vi "Breakdown Point Detection.vi"() -> ()   [LabVIEW 2023]
doc: "This example shows the application of the continuous wavelet transform (CWT) in detecting breakdown points in a signal.\n\nBoth breakdown points and noise can generate large values in the resulting CWT coefficients. Breakdown points generate large positive or negative coefficients at all scales. Noise generates positive coefficients at some scales and negative coefficients at other scales. If you accumulate the coefficients at all scales, the coefficients of breakdown points are enlarged while the coefficients of noise at different scales counteract one another. Therefore, the peaks in the accumulated CWT coefficients correspond only to the breakdown points.\n\nThis example uses the WA Continuous Wavelet Transform VI to compute the CWT coefficients of a simulated signal and use the WA Multiscale Peak Detection VI to detect the peaks in the accumulated CWT coefficients.\n\n<b>Instructions:</b>\n1) Run this VI.\n2) Observe the peaks in the <b>CWT Coefficients Cumulation</b> graph.\n3) Browse the Block Diagram of this example to learn how to detect breakdown points in a signal with the continuous wavelet transform."
uses:
  <vilib>/addons/Wavelet Analysis/typedefs.llb/WA Data.ctl
  <vilib>/addons/Wavelet Analysis/continuous wavelet transform.llb/WA Continuous Wavelet Transform (Array).vi
  <vilib>/addons/Wavelet Analysis/application.llb/WA Multiscale Peak Detection (Array).vi
  <vilib>/addons/_Advanced Signal Processing/NI_AdvSigProcWA.lvlib
  <vilib>/Analysis/NI_AALBase.lvlib
panel:
  in  "stop":bool
  out "CWT Coefficients Cumulation":dbl[](graph)
  out "Breakdown locations":dbl[](array[numeric])
  in  "Noise level":dbl=0.4 min=0.0 step=0.05
  in  "Scales":i32=20 min=2 max=32 step=1
  out "Scalogram":dbl[][](graph)
  out "Signal":dbl[][](graph)
  # "Overview: Shows the application of the continuous wavelet transform (CWT) in detecting breakdown points in a signal.\nRequirements: LabVIEW Full Development System, Advanced Signal Processing Toolkit\nInstructions: \n1. Run this VI.\n2. Observe the peaks in the CWT Coefficients Cumulation graph.\n3. Browse the block diagram of this example to learn how to detect breakdown points in a signal with the continuous wavelet transform.\n4. Click Stop to stop the VI."
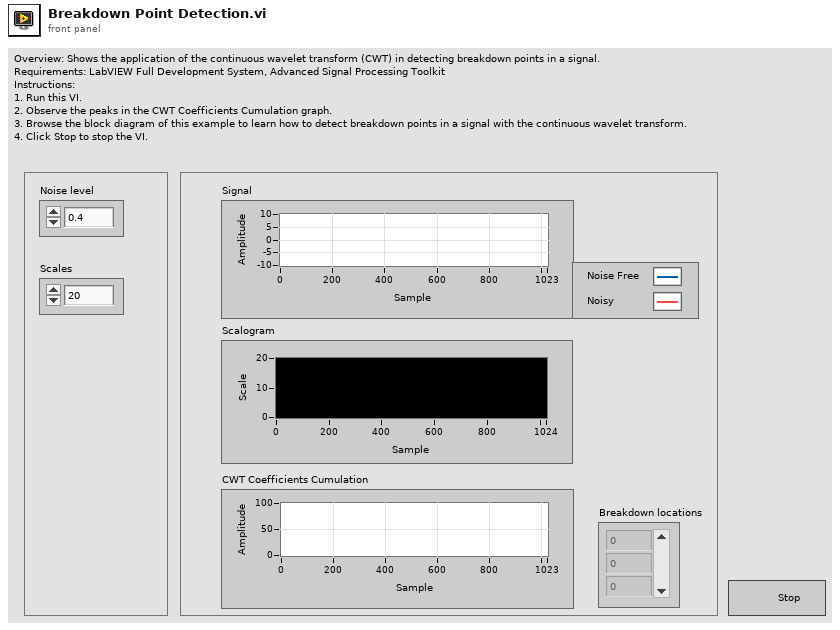
[diagram p1: front panel]
types:
  T1 = typedef "NI_AdvSigProcWA.lvlib/WA Data.ctl" = u16
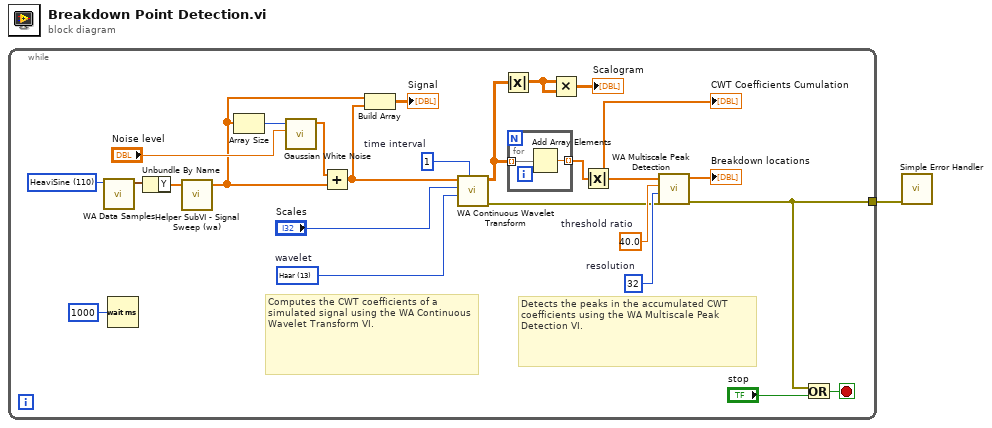
[diagram p0: block diagram]
diagram:
  n1 = while {
    tunnel: [w2] -> w1
    stop <- w10 stop-if-true
    w3 = T1 110 items=["1D Example Data"=100, "-"=101, "Doppler"=102, "HOP"=103, "TF Sine"=104, "Noisy Doppler"=105, "Sea Temperature"=106, "Sp500"=107, "Power Line"=108, "Engine Knocking"=109, "HeaviSine"=110, "Bumps"=111, "Blocks"=112, "Piece Regular"=113, "HypChirps"=114, "LinChirps"=115, "Chirps"=116, "Piece Polynomial"=117, "ECG"=131, "-"=118, "2D Example Data"=119, "-"=120, "Finger Print (Image)"=121, "Iris Flower (Image)"=122, "Mammogram (Image)"=123, "Lake (Image)"=127, "Two Can 1 (Image)"=132, "Two Can 2 (Image)"=133, "Camera Man (Image)"=134] ("data")
    w13 = u16 13 items=["Mexican Hat"=50, "Meyr"=51, "Morlet"=52, "-"=53, "db02"=0, "db03"=1, "db04"=2, "db05"=3, "db06"=4, "db07"=5, "db08"=6, "db09"=7, "db10"=8, "db11"=9, "db12"=10, "db13"=11, "db14"=12, "Haar"=13, "bior1_3"=14, "bior1_5"=15, "bior2_2"=16, "bior2_4"=17, "bior2_6"=18, "bior2_8"=19, "bior3_1"=20, "bior3_3"=21, "bior3_5"=22, "bior3_7"=23, "bior3_9"=24, "bior4_4 (FBI)"=25, "bior5_5"=38, "bior6_8"=39, "coif1"=26, "coif2"=27, "coif3"=28, "coif4"=29, "coif5"=30, "sym2"=31, "sym3"=32, "sym4"=33, "sym5"=34, "sym6"=35, "sym7"=36, "sym8"=37]  # wavelet
    w15 = 32  # resolution
    w16 = 40.0  # threshold ratio
    w25 = 1  # time interval
    # "Detects the peaks in the accumulated CWT coefficients using the WA Multiscale Peak Detection VI."
    # "Computes the CWT coefficients of a simulated signal using the WA Continuous Wavelet Transform VI."
    n2 = call <vilib>:"WA Data Samples.vi"("data"=w3) -> ("signal"=w26:waveform(dbl))  [unwired: 10 out]
    n3 = Wait (ms)(milliseconds to wait=u32 1000 ("millisecond multiple")) -> ()  [unwired: 1 out]
    n4 = Unbundle By Name(w26) -> ("Y"=w8:dbl[])
    n5 = call "Helper SubVI - Signal Sweep (wa).vi"("Signal in"=w8) -> ("Signal out"=w7:dbl[])  [unwired: 10 in]
    n6 = Array Size(array=w7) -> (size(s)=w23:i32)
    n7 = call <vilib>:"Gaussian White Noise.vi"("standard deviation"="Noise level", "samples"=w23) -> ("Gaussian noise pattern"=w22:dbl[])  [unwired: 8 in, 1 out]
    n8 = Add(x=w22, y=w7) -> (x+y=w19:dbl[])
    n9 = Build Array(w7, w19) -> (→"Signal":dbl[][])
    n10 = call-poly <vilib>:"WA Continuous Wavelet Transform.vi"("time steps"=w25, "wavelet"=w13, "scales"="Scales", "signal"=w19) -> ("error out"=w12:errorcluster, "CWT coef"=w6:dbl[][])  [unwired: 1 in, 5 out]
    n11 = Absolute Value(x=w6) -> (abs(x)=w5:dbl[][])
    n12 = for {
      tunnel: w6 -> [w27] mode=indexing
      tunnel: [w28] -> w18 mode=indexing
      n13 = Add Array Elements(numeric array=w27) -> (sum=w28:dbl)
    }
    n14 = Multiply(x=w5, y=w5) -> (x*y=→"Scalogram":dbl[][])
    n15 = Absolute Value(x=w18) -> (abs(x)=w17:dbl[])
    "CWT Coefficients Cumulation" <- w17
    n16 = call-poly <vilib>:"WA Multiscale Peak Detection.vi"("error in (no error)"=w12, "width"=w15, "threshold"=w16, "signal"=w17) -> ("error out"=w2:errorcluster, "location"=→"Breakdown locations":dbl[])  [unwired: 3 in, 3 out]
    n17 = Or(x=w2, y="stop") -> (x .or. y?=w10:bool)
  }
  n18 = call <vilib>:"Simple Error Handler.vi"("error in (no error)"=w1) -> ()  [unwired: 1 in, 8 out]
